vi "test_dualPatch_v02.vi"(4 "experiment day folder":path=path "C:/Users/ikolb3/Dropbox (Personal)/patcherBot/data/9-25-2017", 7 "dual patch cluster":T1={"sampling rate (Hz)"=20000.0, "total duration (s)"=5.0, "stim amplitude (pA)"=2000.0, "time between stims (s)"=3.0, "delta t (s)"=0.01, "pulse width (s)"=0.002, "# repetitions"=3.0, "number of pulses"=10, "before stim (s)"=1.0}, 8 "AO error in":errorcluster, 10 "AI Physical Channel":tag="Dev1/ai0:2, Dev1/ai10", 11 "AO physical channels":tag="Dev1/ao0:1") -> (0 "error out":errorcluster)   [LabVIEW 2015]
uses:
  <vilib>/DAQmx/configure/timing.llb/DAQmx Timing (Sample Clock).vi
  <vilib>/DAQmx/create/channels.llb/DAQmx Create Channel (AI-Voltage-Basic).vi
  <vilib>/DAQmx/create/channels.llb/DAQmx Create Channel (AO-Voltage-Basic).vi
  <vilib>/DAQmx/configure/trigger.llb/DAQmx Start Trigger (Digital Edge).vi
  <vilib>/DAQmx/write.llb/DAQmx Write (Analog 1D Wfm NChan NSamp).vi
  <vilib>/DAQmx/read.llb/DAQmx Read (Analog 1D Wfm NChan NSamp).vi
  <vilib>/Analysis/NI_AALBase.lvlib
  <vilib>/Waveform/WDTOps.llb/WDT Append Waveforms DBL.vi
  controls/dual_patch_controls.ctl
panel:
  out "twitter?":bool
  out "secondary out (pA)":waveform(dbl)[](graph)
  in  "which clamp":enum16{"VClamp", "IClamp"}(ring)=enum."IClamp"
  out "primary out (mV)":waveform(dbl)[](graph)
  in  "AI error in":errorcluster
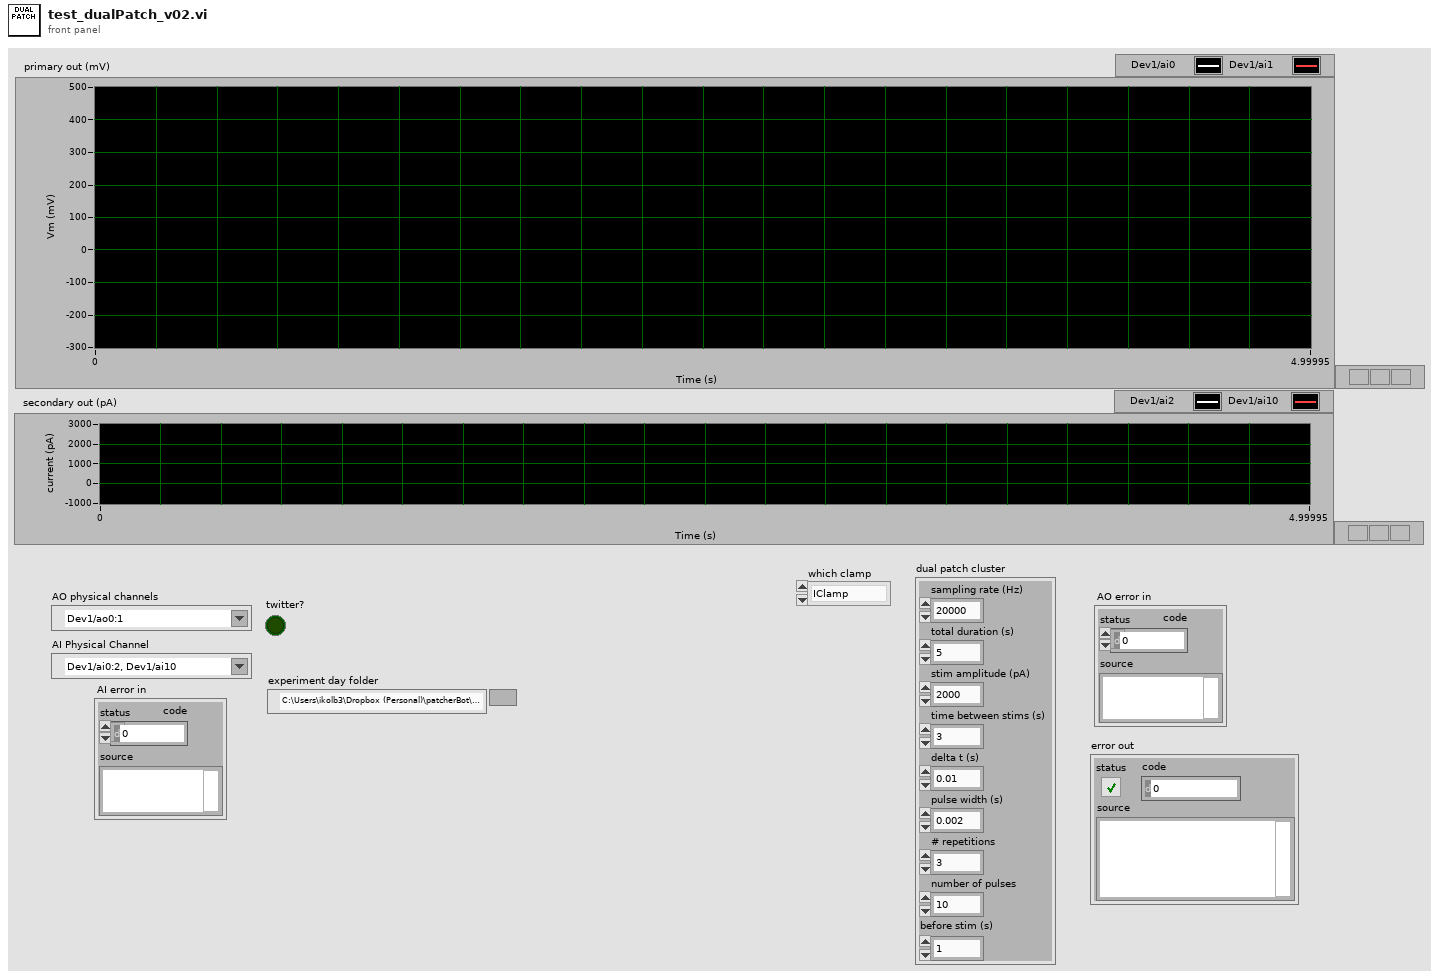
[diagram p1: front panel]
types:
  T1 = typedef "dual_patch_controls.ctl" = cluster{"sampling rate (Hz)":dbl, "total duration (s)":dbl, "stim amplitude (pA)":dbl, "time between stims (s)":dbl, "delta t (s)":dbl, "pulse width (s)":dbl, "# repetitions":dbl, "number of pulses":i32, "before stim (s)":dbl}
  T2 = cluster{"Prototype Pulse":dbl[], "delta t of Prototype Pulse (s) ":dbl}
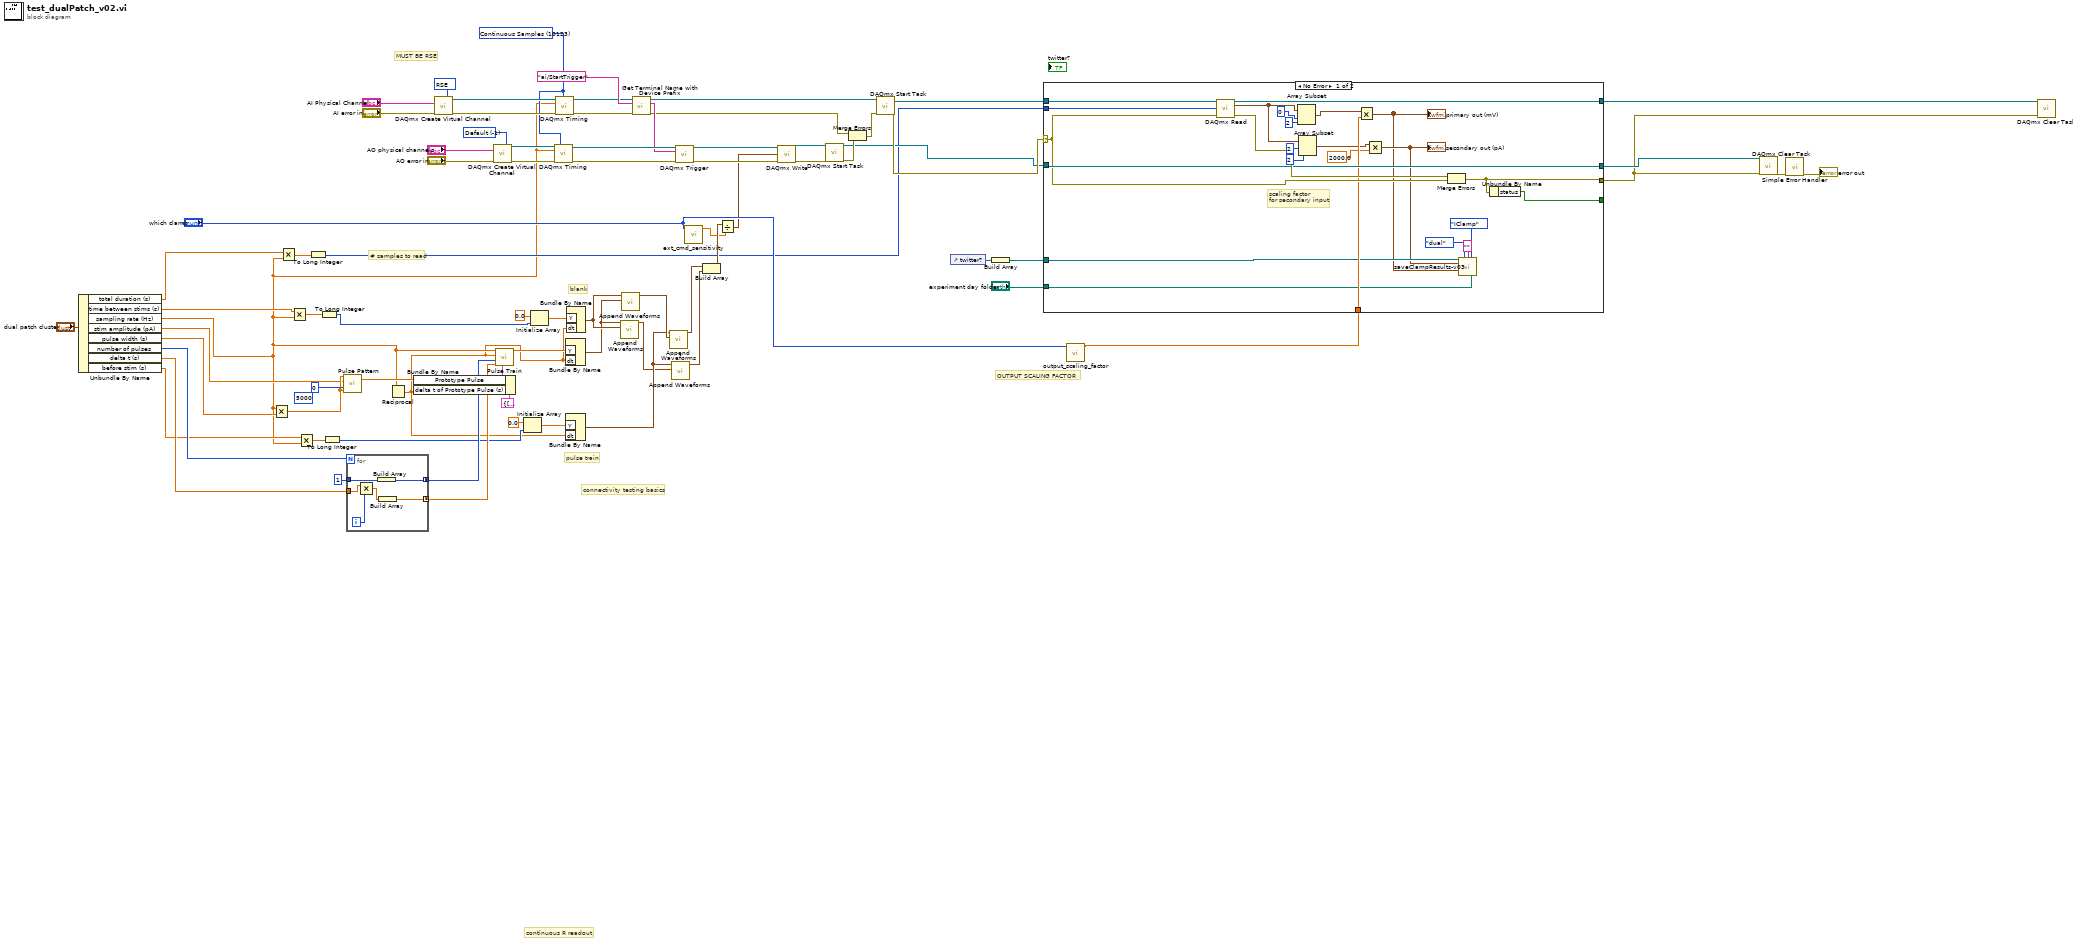
[diagram p0: block diagram]
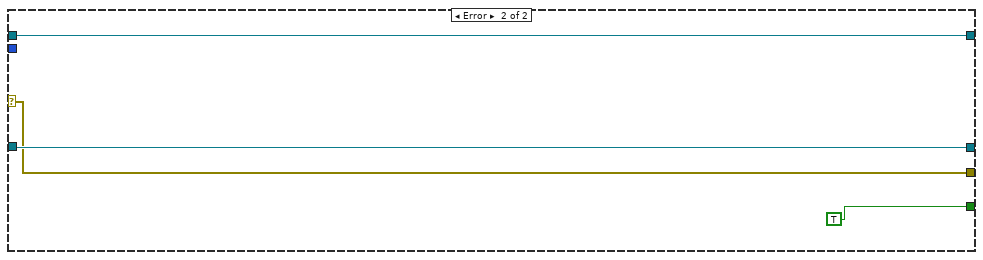
[diagram p2: hidden frame]
diagram:
  w35 = -1 items=["Default"=-1, "RSE"=10083, "Differential"=10106, "Pseudodifferential"=12529] ("output terminal configuration")
  (unwired) 5000 ("width")
  w74 = 10083 items=["default"=-1, "RSE"=10083, "NRSE"=10078, "Differential"=10106, "Pseudodifferential"=12529] ("input terminal configuration")
  w65 = 10123 items=["Finite Samples"=10178, "Continuous Samples"=10123] ("sample mode")
  # "# samples to read"
  # "connectivity testing basics"
  # "MUST BE RSE"
  # "pulse train"
  # "blank"
  # "OUTPUT SCALING FACTOR"
  # "continuous R readout"
  n1 = Unbundle By Name("dual patch cluster") -> ("total duration (s)"=w21:dbl, "time between stims (s)"=w20:dbl, "sampling rate (Hz)"=w12:dbl, "stim amplitude (pA)"=w18:dbl, "pulse width (s)"=w19:dbl, "number of pulses"=w17:i32, "delta t (s)"=w16:dbl, "before stim (s)"=w13:dbl)
  n2 = Multiply(x=w12, y=w19) -> (x*y=w28:dbl)
  n3 = Multiply(x=w21, y=w12) -> (x*y=w27:dbl)
  n4 = Multiply(x=w20, y=w12) -> (x*y=w25:dbl)
  n5 = Multiply(x=w13, y=w12) -> (x*y=w14:dbl)
  n6 = To Long Integer(number=w27) -> (32bit integer=w26:i32)
  n7 = To Long Integer(number=w25) -> (32bit integer=w24:i32)
  n8 = To Long Integer(number=w14) -> (32bit integer=w11:i32)
  n9 = call <vilib>:"Pulse Pattern.vi"("width"=w28, "delay"=0, "amplitude"=w18, "samples"=w28) -> ("Pulse Pattern"=w42:dbl[])  [unwired: 1 out]
  n10 = for {
    N: w17 -> [_]
    tunnel: 1 -> [w82]
    tunnel: [w83] -> w30 mode=concatenating
    tunnel: w16 -> [w79]
    tunnel: [w80] -> w29 mode=concatenating
    i -> [w78]
    n11 = Multiply(x=w79, y=w78) -> (x*y=w81:dbl)
    n12 = Build Array(w82) -> (w83:i32[])
    n13 = Build Array(w81) -> (w80:dbl[])
  }
  n14 = Reciprocal(x=w12) -> (1/x=w9:dbl)
  n15 = Bundle By Name(cluster=T2 {"Prototype Pulse"=[], "delta t of Prototype Pulse (s) "=0.1} ("prototype spec"), "Prototype Pulse"=w42, "delta t of Prototype Pulse (s)"=w9) -> (w45:T2)
  n16 = call-poly <vilib>:"DAQmx Create Virtual Channel.vi"("input terminal configuration"=w74, "physical channels"="AI Physical Channel", "error in"="AI error in") -> ("task out"=w76:refnum<k21>, "error out"=w77:errorcluster)  [unwired: 11 in]
  n17 = call-poly <vilib>:"DAQmx Create Virtual Channel.vi"("output terminal configuration"=w35, "physical channels"="AO physical channels", "error in"="AO error in") -> ("task out"=w67:refnum<k21>, "error out"=w66:errorcluster)  [unwired: 11 in]
  n18 = call <vilib>:"Pulse Train.vi"("prototype spec"=w45, "Delay (s)"=w29, "Amplitude"=w30, "delta t of pulse train (s)"=w9, "samples"=w12) -> ("Pulse Train"=w41:dbl[])  [unwired: 5 in, 1 out]
  n19 = Initialize Array(0.0 ("element"), w11) -> (w10:dbl[])
  n20 = Initialize Array(0.0 ("element"), w24) -> (w39:dbl[])
  n21 = call-poly <vilib>:"DAQmx Timing.vi"("task/channels in"=w67, "sample mode"=w65, "rate"=w12, "error in"=w66) -> ("task out"=w63:refnum<k21>, "error out"=w64:errorcluster)  [unwired: 10 in]
  n22 = call-poly <vilib>:"DAQmx Timing.vi"("task/channels in"=w76, "sample mode"=w65, "rate"=w12, "error in"=w77) -> ("task out"=w71:refnum<k21>, "error out"=w70:errorcluster)  [unwired: 10 in]
  n23 = Bundle By Name("Y"=w41, "dt"=w9) -> (w36:waveform(dbl))  [unwired: 1 in]
  n24 = Bundle By Name("Y"=w10, "dt"=w9) -> (w7:waveform(dbl))  [unwired: 1 in]
  n25 = Bundle By Name("Y"=w39, "dt"=w9) -> (w37:waveform(dbl))  [unwired: 1 in]
  n26 = call-poly <vilib>:"Append Waveforms.vi"("waveform B"=w37, "waveform A"=w36) -> ("waveform out"=w6:waveform(dbl))  [unwired: 8 in, 1 out]
  n27 = call-poly <vilib>:"Append Waveforms.vi"("waveform B"=w36, "waveform A"=w37) -> ("waveform out"=w8:waveform(dbl))  [unwired: 8 in, 1 out]
  n28 = call "Get Terminal Name with Device Prefix.vi"("error in (no error)"=w70, "Local Terminal Name"="ai/StartTrigger" ("terminal"), "task/channels in"=w71) -> ("error out"=w59:errorcluster, "Terminal Name with Device Prefix"=w62:tag, "task out"=w54:refnum<k21>)  [unwired: 6 in]
  n29 = call-poly <vilib>:"Append Waveforms.vi"("waveform B"=w8, "waveform A"=w7) -> ("waveform out"=w1:waveform(dbl))  [unwired: 8 in, 1 out]
  n30 = call-poly <vilib>:"Append Waveforms.vi"("waveform B"=w6, "waveform A"=w7) -> ("waveform out"=w5:waveform(dbl))  [unwired: 8 in, 1 out]
  n31 = call-poly <vilib>:"DAQmx Trigger.vi"("task/channels in"=w63, "source"=w62, "error in"=w64) -> ("task out"=w61:refnum<k21>, "error out"=w60:errorcluster)  [unwired: 11 in]
  n32 = call "ext_cmd_sensitivity.vi"("which clamp"="which clamp") -> ("division factor"=w33:dbl)  [unwired: 10 in]
  n33 = Build Array(w1, w5) -> (w34:waveform(dbl)[])
  n34 = Divide(x=w34, y=w33) -> (x/y=w23:waveform(dbl)[])
  n35 = call-poly <vilib>:"DAQmx Write.vi"("task/channels in"=w61, "data"=w23, "error in"=w60) -> ("task out"=w56:refnum<k21>, "error out"=w55:errorcluster)  [unwired: 10 in, 1 out]
  n36 = call <vilib>:"DAQmx Start Task.vi"("task/channels in"=w56, "error in"=w55) -> ("task out"=w51:refnum<k21>, "error out"=w57:errorcluster)  [unwired: 12 in]
  n37 = Merge Errors(w59, w57) -> (w58:errorcluster)
  n38 = call <vilib>:"DAQmx Start Task.vi"("task/channels in"=w54, "error in"=w58) -> ("task out"=w53:refnum<k21>, "error out"=w52:errorcluster)  [unwired: 12 in]
  n39 = control-ref of="twitter?"() -> (w4:refnum<vi>)
  n40 = Build Array(w4) -> (w3:refnum<vi>[])
  n41 = call "output_scaling_factor.vi"("which clamp"="which clamp") -> ("output scaling factor"=w38:dbl)  [unwired: 10 in]
  n42 = case shown="No Error" w52 {
    selector: w52 -> [w104 w108]
    tunnel: w53 -> [w107 w110]
    tunnel: w51 -> [w105 w109]
    tunnel: [w102 TRUE ("status")] -> _
    tunnel: [w105 w109] -> w49
    tunnel: [w94 w110] -> w50
    tunnel: [w103 w108] -> w48
    tunnel: w38 -> [w101 _]
    tunnel: w26 -> [w91 _]
    tunnel: w3 -> [w88 _]
    tunnel: "experiment day folder" -> [w87 _]
    frame No Error {
      # "scaling factor\nfor secondary input"
      n43 = call-poly <vilib>:"DAQmx Read.vi"("task/channels in"=w107, "number of samples per channel"=w91, "error in"=w104) -> ("task out"=w94:refnum<k21>, "data"=w97:waveform(dbl)[], "error out"=w106:errorcluster)  [unwired: 10 in]
      n44 = Array Subset(array=w97, index=0, length=2) -> (w98:waveform(dbl)[])
      n45 = Array Subset(array=w97, index=2, length=2) -> (w93:waveform(dbl)[])
      n46 = Multiply(x=w98, y=w101) -> (x*y=w85:waveform(dbl)[])
      "primary out (mV)" <- w85
      n47 = Multiply(x=w93, y=2000.0) -> (x*y=w86:waveform(dbl)[])
      "secondary out (pA)" <- w86
      n48 = Merge Errors(w106, w104) -> (w103:errorcluster)
      n49 = call "saveClampResults-v03.vi"("controls array"=w88, "protocol or memtest"=enum16{"protocol", "memtest", "dual"}."dual", "ExpPhase"="", "which clamp"=enum16{"VClamp", "IClamp"}."IClamp", "view profile"=w86, "rec profile"=w85, "Save to (folder dir)"=w87) -> ()  [unwired: 7 in, 2 out]
      n50 = Unbundle By Name(w103) -> ("status"=w102:bool)
    }
    frame Error {
    }
  }
  n51 = call <vilib>:"DAQmx Clear Task.vi"("task in"=w49, "error in"=w48) -> ("error out"=w47:errorcluster)  [unwired: 13 in]
  n52 = call <vilib>:"Simple Error Handler.vi"("error in (no error)"=w47) -> ("error out"=→"error out":errorcluster)  [unwired: 4 in, 4 out]
  n53 = call <vilib>:"DAQmx Clear Task.vi"("task in"=w50, "error in"=w48) -> ()  [unwired: 13 in, 1 out]
